vi "RebuildCmdListing.vi"(3 "Params":cluster{"Constant":string, "value":string}[](array[cluster]), 4 "Contents":string, 5 "String in":string) -> (1 "array":string[](array[string]), 2 "String out":string)   [LabVIEW 2012]
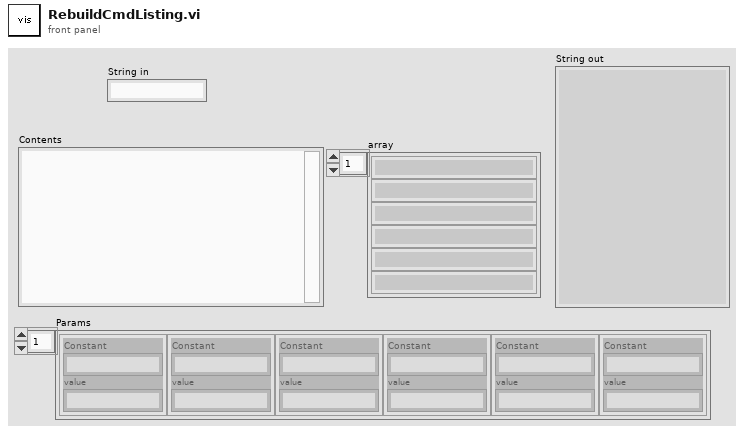
[diagram p1: front panel]
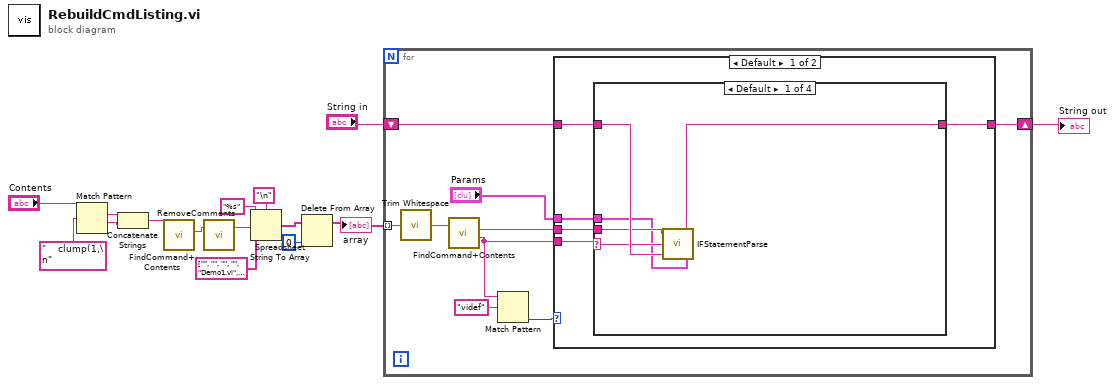
[diagram p0: block diagram]
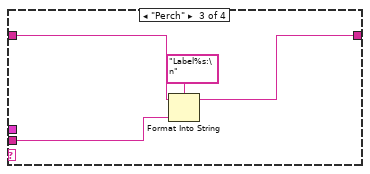
[diagram p3: hidden frame]
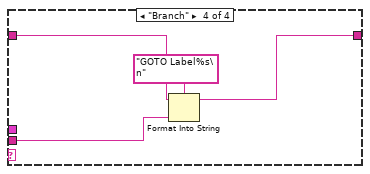
[diagram p4: hidden frame]
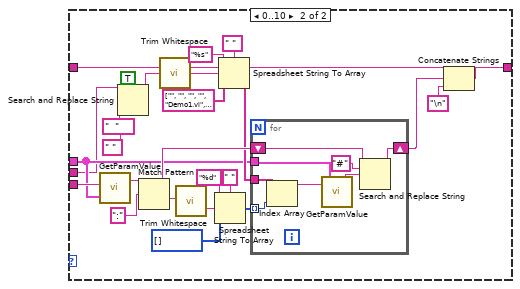
[diagram p5: hidden frame]
diagram:
  n1 = Match Pattern(string="Contents", regular expression="    clump(1,\n") -> (match substring=w7:string, after substring=w8:string)  [unwired: 1 in, 2 out]
  n2 = Concatenate Strings(w7, w8) -> (w9:string)
  n3 = call "FindCommand+Contents.vi"("Via file in"=w9) -> ("Contents"=w10:string)  [unwired: 1 in, 3 out]
  n4 = call "RemoveComments.vi"("Via file in"=w10) -> ("Via file out"=w11:string)  [unwired: 2 in]
  n5 = Spreadsheet String To Array(delimiter (Tab)="\n", format string="%s", spreadsheet string=w11, array type (2D Dbl)=string[] ["", "", "", "", "Demo1.vi", "DigitalWrite.vi", "VS_Wait.vi", ""] ("Array 3")) -> (array=w14:string[])
  n6 = Delete From Array(array=w14, index=0) -> (array with subset deleted=w3:string[])  [unwired: 1 in, 1 out]
  "array" <- w3
  n7 = for {
    tunnel: w3 -> [w24] mode=indexing
    shift-right: [w21] -> w2
    shift-left: "String in" -> [w22]
    n8 = call <vilib>:"Trim Whitespace.vi"("string"=w24) -> ("trimmed string"=w23:string)  [unwired: 1 in]
    n9 = call "FindCommand+Contents.vi"("Via file in"=w23) -> ("Contents"=w19:string, "command"=w18:string)  [unwired: 1 in, 2 out]
    n10 = Match Pattern(string=w18, regular expression="videf") -> (offset past match=w16:i32)  [unwired: 1 in, 3 out]
    n11 = case shown="Default" w16 {
      tunnel: w18 -> [w29 w68]
      tunnel: w22 -> [w28 w55]
      tunnel: [w26 w54] -> w21
      tunnel: "Params" -> [w25 w51]
      tunnel: w19 -> [w27 w48]
      frame Default {
        n12 = case shown="Default" w29 {
          selector: w29 -> [w32 _ _ _]
          tunnel: w28 -> [w34 w35 w38 w42]
          tunnel: w27 -> [w33 _ w37 w41]
          tunnel: [w31 w35 w36 w40] -> w26
          tunnel: w25 -> [w30 _ _ _]
          frame Default {
            n13 = call "IFStatementParse.vi"("Params"=w30, "BotSpeak in"=w34, "Command"=w32, "Contents"=w33) -> ("BotSpeak out"=w31:string)  [unwired: 1 in]
          }
          frame "" {
          }
          frame "Perch" {
            n14 = Format Into String(format string="Label%s:\n", initial string=w38, w37) -> (resulting string=w36:string)  [unwired: 1 in, 1 out]
          }
          frame "Branch" {
            n15 = Format Into String(format string="GOTO Label%s\n", initial string=w42, w41) -> (resulting string=w40:string)  [unwired: 1 in, 1 out]
          }
        }
      }
      frame 0..10 {
        n16 = call "GetParamValue.vi"("Params"=w51, "command"=w68) -> ("value"=w67:string)  [unwired: 1 in]
        n17 = Search and Replace String(replace all?=TRUE ("replace all? (F)"), input string=w48, search string="  ", replace string=" " ("replace string (\"\")")) -> (result string=w44:string)  [unwired: 4 in, 3 out]
        n18 = Match Pattern(string=w67, regular expression=":") -> (before substring=w58:string, after substring=w65:string)  [unwired: 1 in, 2 out]
        n19 = call <vilib>:"Trim Whitespace.vi"("string"=w44) -> ("trimmed string"=w49:string)  [unwired: 1 in]
        n20 = call <vilib>:"Trim Whitespace.vi"("string"=w65) -> ("trimmed string"=w50:string)  [unwired: 1 in]
        n21 = Spreadsheet String To Array(delimiter (Tab)=" ", format string="%d", spreadsheet string=w50, array type (2D Dbl)=i32[] [] ("Array 3")) -> (array=w56:i32[])
        n22 = Spreadsheet String To Array(delimiter (Tab)=" ", format string="%s", spreadsheet string=w49, array type (2D Dbl)=string[] ["", "", "", "", "Demo1.vi", "DigitalWrite.vi", "VS_Wait.vi", ""] ("Array 3")) -> (array=w57:string[])
        n23 = for {
          shift-right: [w75] -> w53
          shift-left: w58 -> [w76]
          tunnel: w57 -> [w73]
          tunnel: w56 -> [w72] mode=indexing
          tunnel: w51 -> [w71]
          n24 = Index Array(array=w73, index=w72) -> (element=w70:string)
          n25 = call "GetParamValue.vi"("Params"=w71, "command"=w70) -> ("value"=w69:string)  [unwired: 1 in]
          n26 = Search and Replace String(input string=w76, search string="#", replace string=w69) -> (result string=w75:string)  [unwired: 5 in, 3 out]
        }
        n27 = Concatenate Strings(w55, w53, "\n" ("delimiter (Tab)")) -> (w54:string)
      }
    }
  }
  "String out" <- w2
